vi "path.expand-vis.vi"(8 "error in (no error)":errorcluster, 11 "Target Path":path) -> (0 "error out":errorcluster, 3 "All Files in Dir":path[](array[path]))   [LabVIEW 2020]
uses:
  99a5df05-d702-44bc-af2b-b74c5eae20a9.vi
  <vilib>/Comparison/Equal/Equal Functor/Equal Functor.lvclass
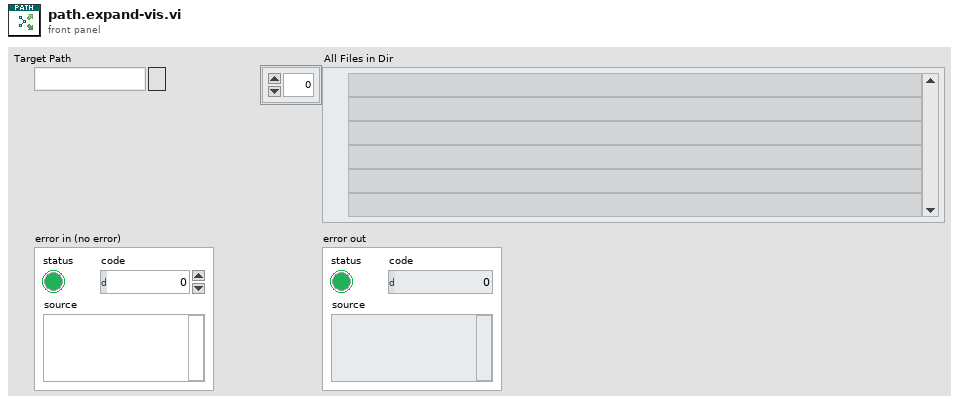
[diagram p1: front panel]
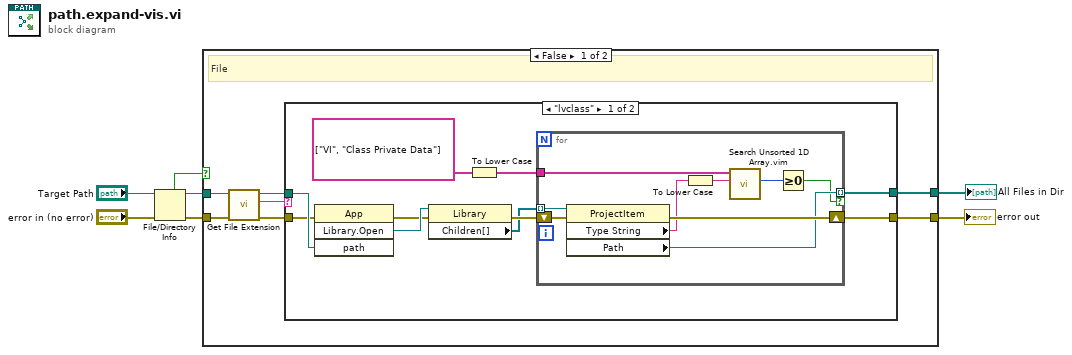
[diagram p0: block diagram]
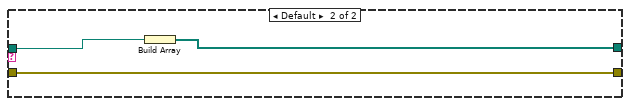
[diagram p2: hidden frame]
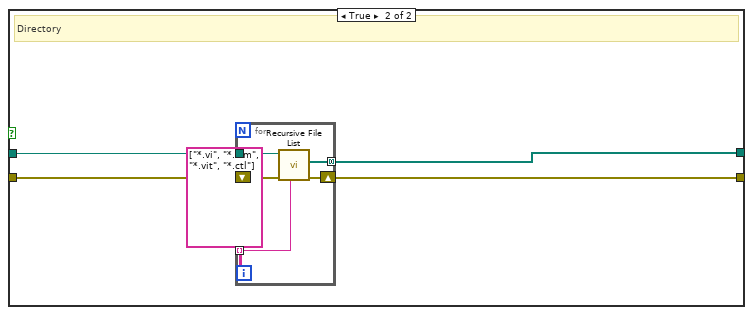
[diagram p3: hidden frame]
diagram:
  n1 = File/Directory Info(path="Target Path", error in="error in (no error)") -> (path out=w2:path, directory=w1:bool, error out=w4:errorcluster)  [unwired: 4 out]
  n2 = case shown="False" w1 {
    tunnel: [w14 w40] -> w7
    tunnel: [w8 w39] -> w6
    tunnel: w4 -> [w13 w38]
    tunnel: w2 -> [w11 w37]
    frame False {
      # "File"
      n3 = call <vilib>:"Get File Extension.vi"("error in (no error)"=w13, "file"=w11) -> ("error out"=w9:errorcluster, "lowercase file extension"=w10:string, "dup file"=w12:path)  [unwired: 5 in, 2 out]
      n4 = case shown="\"lvclass\"" w10 {
        tunnel: [w15 w36] -> w14
        tunnel: w12 -> [w24 w35]
        tunnel: w9 -> [w23 w34]
        tunnel: [w18 w34] -> w8
        frame "lvclass" {
          n5 = invoke class="App" method="Library.Open"(error in=w23, "path"=w24) -> (error out=w21:errorcluster, "Open Library"=w22:refnum<vi>)  [unwired: 2 in, 2 out]
          n6 = property class="Library"(reference=w22, error in=w21) -> (error out=w20:errorcluster, "Children[]"=w19:refnum<vi>[])  [unwired: 1 out]
          n7 = To Lower Case(string=string[] ["VI", "Class Private Data"]) -> (all lower case string=w16:string[])
          n8 = for {
            tunnel: w19 -> [w32] mode=indexing
            shift-right: [w31] -> w18
            shift-left: w20 -> [w33]
            tunnel: w16 -> [w30]
            tunnel: [w28] -> w15 mode=indexing if=w26
            n9 = property class="ProjectItem"(reference=w32, error in=w33) -> (error out=w31:errorcluster, "Type String"=w25:string, "Path"=w28:path)  [unwired: 1 out]
            n10 = To Lower Case(string=w25) -> (all lower case string=w29:string)
            n11 = call "Search Unsorted 1D Array.vim"("element"=w29, "unsorted 1D array"=w30) -> ("index of element"=w27:i32)  [unwired: 9 in]
            n12 = Greater Or Equal To 0?(x=w27) -> (x >= 0?=w26:bool)
          }
        }
        frame Default {
          n13 = Build Array(w35) -> (w36:path[])
        }
      }
    }
    frame True {
      # "Directory"
      n14 = for {
        tunnel: [w45] -> w40 mode=concatenating
        tunnel: w37 -> [w44]
        tunnel: string[] ["*.vi", "*.vim", "*.vit", "*.ctl"] ("pattern") -> [w42] mode=indexing
        shift-right: [w46] -> w39
        shift-left: w38 -> [w43]
        n15 = call <vilib>:"Recursive File List.vi"("pattern"=w42, "error in (no error)"=w43, "Folder Path"=w44) -> ("error out"=w46:errorcluster, "All Files in Dir"=w45:path[])  [unwired: 4 in, 3 out]
      }
    }
  }
  "All Files in Dir" <- w7
  "error out" <- w6
